vi "Check-speed.vi"(8 "error in (no error)":errorcluster, 10 "Speed in":dbl, 11 "Motor in":refnum<class "Motor.lvclass">) -> (0 "error out":errorcluster, 1 "In range?":bool, 2 "Speed out":dbl, 3 "Motor out":refnum<class "Motor.lvclass">)   [LabVIEW 2013, in "PowderDeposition.lvlib" / "Motor.lvclass"]
uses:
  Motor.lvclass
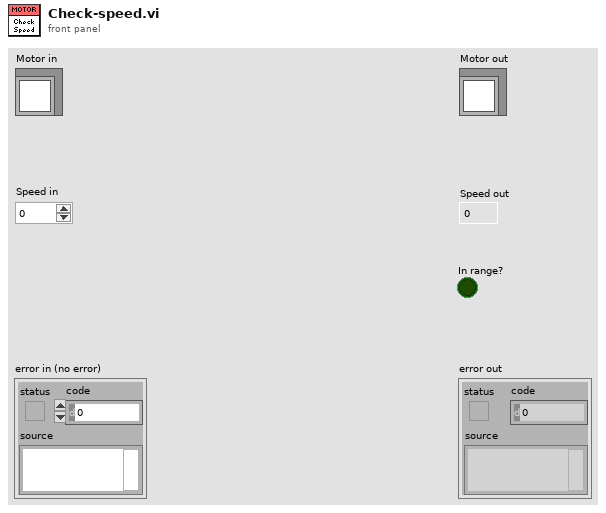
[diagram p1: front panel]
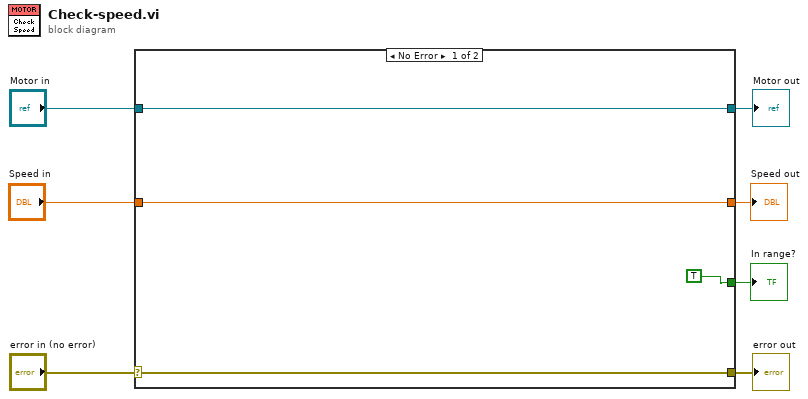
[diagram p0: block diagram]
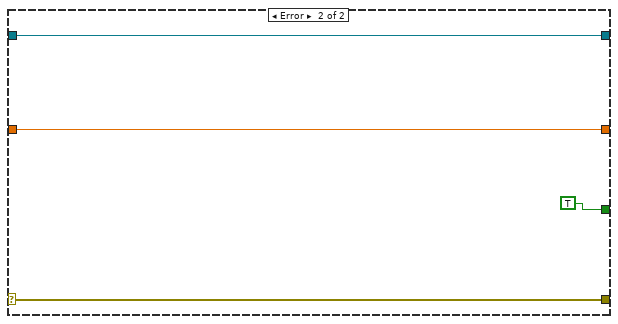
[diagram p2: hidden frame]
diagram:
  n1 = case shown="No Error" "error in (no error)" {
    selector: "error in (no error)" -> [w10 w15]
    tunnel: [w10 w15] -> w6
    tunnel: [w11 w14] -> w4
    tunnel: "Motor in" -> [w11 w14]
    tunnel: "Speed in" -> [w9 w13]
    tunnel: [w9 w13] -> w2
    tunnel: [TRUE TRUE] -> w1
    frame No Error {
    }
    frame Error {
    }
  }
  "error out" <- w6
  "Motor out" <- w4
  "Speed out" <- w2
  "In range?" <- w1
